vi "IMAQ LL-Grab.vi"(8 "ErrIn":errorcluster, 11 "IF Name":string="img0") -> (0 "ErrOut":errorcluster, 3 "ImgOut":T1)   [LabVIEW 2013]
doc: "Use this template to build a VI to use as a subVI."
uses:
  <vilib>/vision/Image Controls.llb/IMAQ Image.ctl
panel:
  in  "stop":bool
  out "Frame Rate":dbl
  # "Input Parameters"
  # "Output Parameters"
  # "VI Description:\nThis VI is created to snap a image from imaging device."
  # ":: MVI Framework V1.0 ::\nAuthor:Gaoke Yang\nEmail: gaoke.yang@yahoo.com\nWeb: www.mvicontrol.com\nCopyright (C) 2013, MVI Technologies All Rights Reserved"
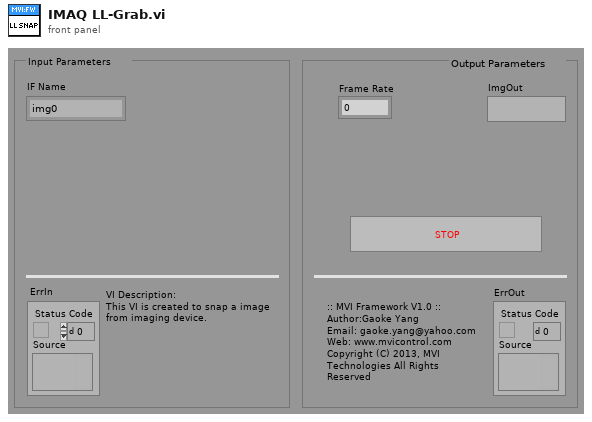
[diagram p1: front panel]
types:
  T1 = typedef "IMAQ Image.ctl" = refnum<image>
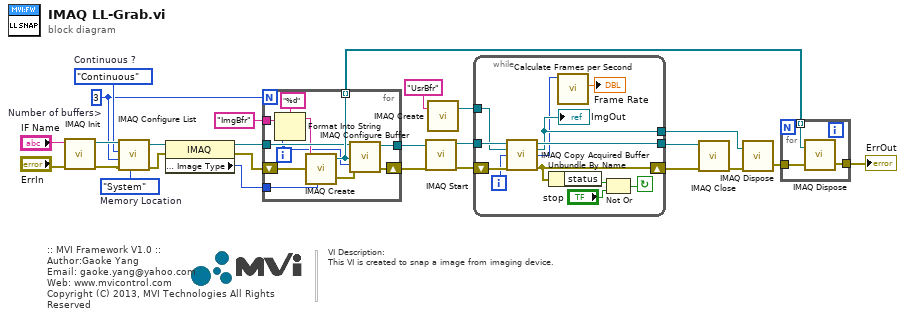
[diagram p0: block diagram]
diagram:
  w21 = enum16{"System", "Onboard"}."System"  # Memory Location
  w5 = u32 3  # Number of buffers>
  w23 = enum16{"One-Shot", "Continuous"}."Continuous"  # Continuous ?
  # "VI Description:\nThis VI is created to snap a image from imaging device."
  # ":: MVI Framework V1.0 ::\nAuthor:Gaoke Yang\nEmail: gaoke.yang@yahoo.com\nWeb: www.mvicontrol.com\nCopyright (C) 2013, MVI Technologies All Rights Reserved"
  n1 = call <vilib>:"IMAQ Init.vi"("error in (no error)"="ErrIn", "Interface Name"="IF Name") -> ("error out"=w22:errorcluster, "IMAQ Session Out"=w24:refnum<k11>)  [unwired: 8 out]
  n2 = call <vilib>:"IMAQ Configure List.vi"("Memory Location"=w21, "error in (no error)"=w22, "Number of buffers"=w5, "Continuous?"=w23, "IMAQ Session In"=w24) -> ("error out"=w19:errorcluster, "IMAQ Session Out"=w20:refnum<k11>)  [unwired: 1 in, 4 out]
  n3 = property class="IMAQ"(reference=w20, error in=w19) -> (reference out=w8:refnum<k11>, error out=w10:errorcluster, "Image Parameters : Image Type"=w4:u32)
  n4 = for {
    N: w5 -> [_]
    tunnel: [w37] -> w7
    tunnel: w4 -> [w35]
    tunnel: w8 -> [w31]
    tunnel: [w32] -> w1 mode=indexing
    shift-right: [w36] -> w9
    shift-left: w10 -> [w34]
    tunnel: "ImgBfr" ("ImgBfr") -> [w27]
    i -> [w29]
    n5 = Format Into String(format string="%d", initial string=w27, w29) -> (resulting string=w30:string)  [unwired: 1 in, 1 out]
    n6 = call "IMAQ Create"("Image Name"=w30, "Image Type"=w35, "error in (no error)"=w34) -> ("New Image"=w32:T1, "error out"=w33:errorcluster)  [unwired: 1 in, 1 out]
    n7 = call <vilib>:"IMAQ Configure Buffer.vi"("error in (no error)"=w33, "Buffer Number"=w29, "Image In"=w32, "IMAQ Session In"=w31) -> ("error out"=w36:errorcluster, "IMAQ Session Out"=w37:refnum<k11>)  [unwired: 2 in, 4 out]
  }
  n8 = call <vilib>:"IMAQ Start.vi"("error in (no error)"=w9, "IMAQ Session In"=w7) -> ("error out"=w11:errorcluster, "IMAQ Session Out"=w12:refnum<k11>)  [unwired: 8 out]
  n9 = call "IMAQ Create"("Image Name"="UsrBfr") -> ("New Image"=w13:T1)  [unwired: 3 in, 2 out]
  n10 = while {
    shift-left: w11 -> [w47]
    shift-right: [w43] -> w16
    tunnel: [w48] -> w18
    tunnel: w12 -> [w49]
    tunnel: [w41] -> w14
    tunnel: w13 -> [w42]
    i -> [w38]
    stop <- w44 continue-if-true
    n11 = call <vilib>:"IMAQ Copy Acquired Buffer.vi"("IMAQ Session In"=w49, "Image In"=w42, "Buffer Number"=w38, "error in (no error)"=w47) -> ("IMAQ Session Out"=w48:refnum<k11>, "Image Out"=w41:T1, "Buffer Number Copied"=w40:i32, "error out"=w43:errorcluster)  [unwired: 2 in, 6 out]
    "ImgOut" <- w41
    n12 = Unbundle By Name(w43) -> ("status"=w46:bool)
    n13 = call <vilib>:"Calculate Frames per Second.vi"("Buffer Number"=w40) -> ("Processed Frames/s"=→"Frame Rate":dbl)  [unwired: 8 in, 2 out]
    n14 = Not Or(1:"stop", 2:w46) -> (0:w44:bool)
  }
  n15 = call <vilib>:"IMAQ Close.vi"("error in (no error)"=w16, "IMAQ Session In"=w18) -> ("error out"=w15:errorcluster)  [unwired: 9 out]
  n16 = call "IMAQ Dispose"("Image"=w14, "error in (no error)"=w15) -> ("error out"=w3:errorcluster)  [unwired: 1 in, 3 out]
  n17 = for {
    tunnel: w1 -> [w52] mode=indexing
    tunnel: [w50] -> w2
    tunnel: w3 -> [w51]
    n18 = call "IMAQ Dispose"("Image"=w52, "error in (no error)"=w51) -> ("error out"=w50:errorcluster)  [unwired: 1 in, 3 out]
  }
  "ErrOut" <- w2
